vi "OceanOptics_30sec_img_while_scan_bare_Minimum.vi"() -> ()   [LabVIEW 2016]
uses:
  Maya2000 Typedefs/Maya2000 basic info.ctl
  C:/Program Files/Ocean Optics/OmniDriver/OOI_HOME/NETOmniDriver-NET40.dll
  Program Files/Ocean Optics/OmniDriver/OOI_HOME/NETOmniDriver-NET40.dll
  <vilib>/DAQmx/write.llb/DAQmx Write (Digital Bool 1Line 1Point).vi
  <vilib>/DAQmx/create/channels.llb/DAQmx Create Channel (DO-Digital Output).vi
  <vilib>/DAQmx/miscellaneous.llb/DAQmx Fill In Error Info.vi
panel:
  out "getExternalTriggerMode 2":i32
  in  "Trigger mode 2":i32
  in  "error in":errorcluster
  out "error out 2":errorcluster
  in  "Trigger":bool
  in  "Action B":bool
  out "getBufferCapacity":i32
  in  "read":bool
  in  "start":bool
  in  "abort":bool
  in  "stop":bool
  out "spectrum":cluster{"Y":dbl[], "Y":dbl[]}[](graph)
  out "getExternalTriggerMode":i32
  in  "Trigger mode":i32
  out "isFeatureSupportedDataBuffer":i16
  in  "clear":bool
  out "getNumberOfElements before readout":i32
  out "status":bool
  out "error out":errorcluster
  out "this maya":T1={"This instruments index"=0, "Name+SerialNumber"="MayaPro2000:MAYP111403", "Number Dark pixels"=8, "NumberOfPixels\nper spectrum"=2068, "NumberOf Maya2000 instrm."=2, "MaximumIntegrationTime\n[us]"=1600000000, "MinimumIntegrationTime\n[us]"=7200}
  in  "integration time [us]":i32=100000
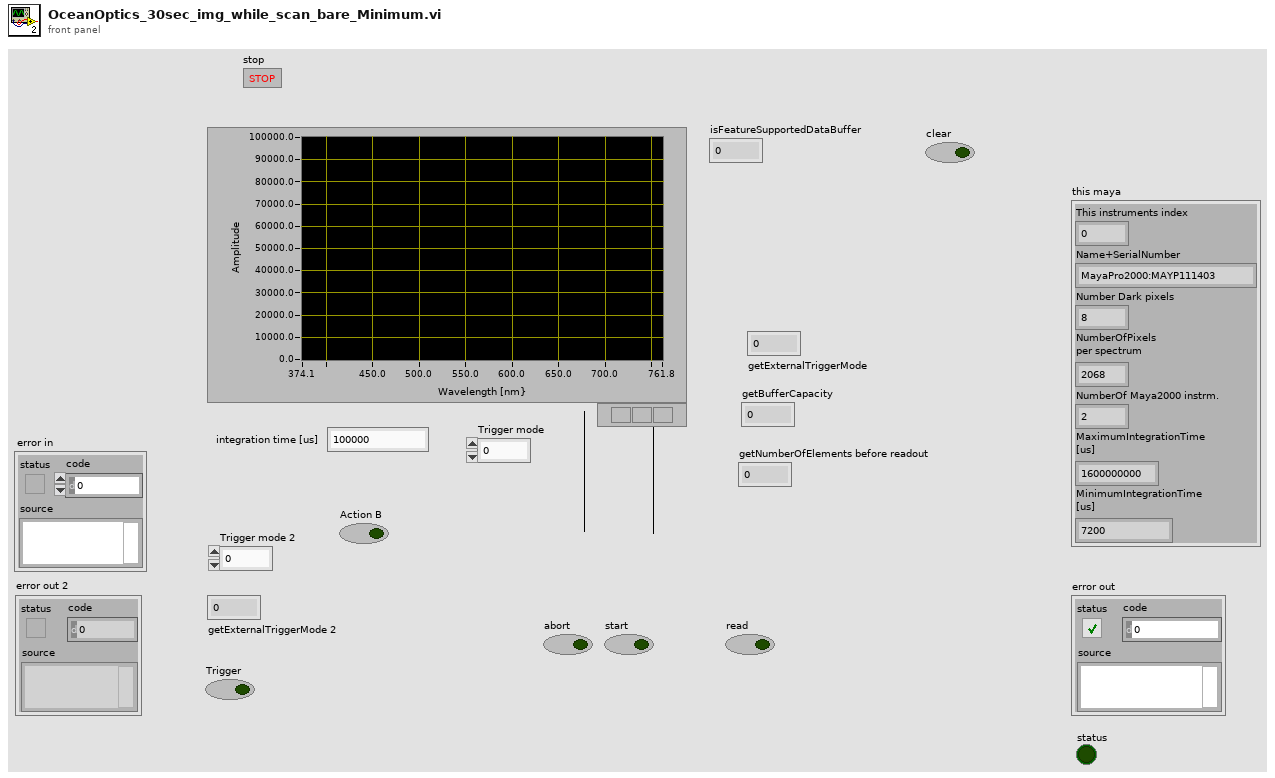
[diagram p1: front panel]
types:
  T1 = typedef "Maya2000 basic info.ctl" = cluster{"This instruments index":i32, "Name+SerialNumber":string, "Number Dark pixels":i32, "NumberOfPixels\nper spectrum":i32, "NumberOf Maya2000 instrm.":i32, "MaximumIntegrationTime\n[us]":i32, "MinimumIntegrationTime\n[us]":i32}
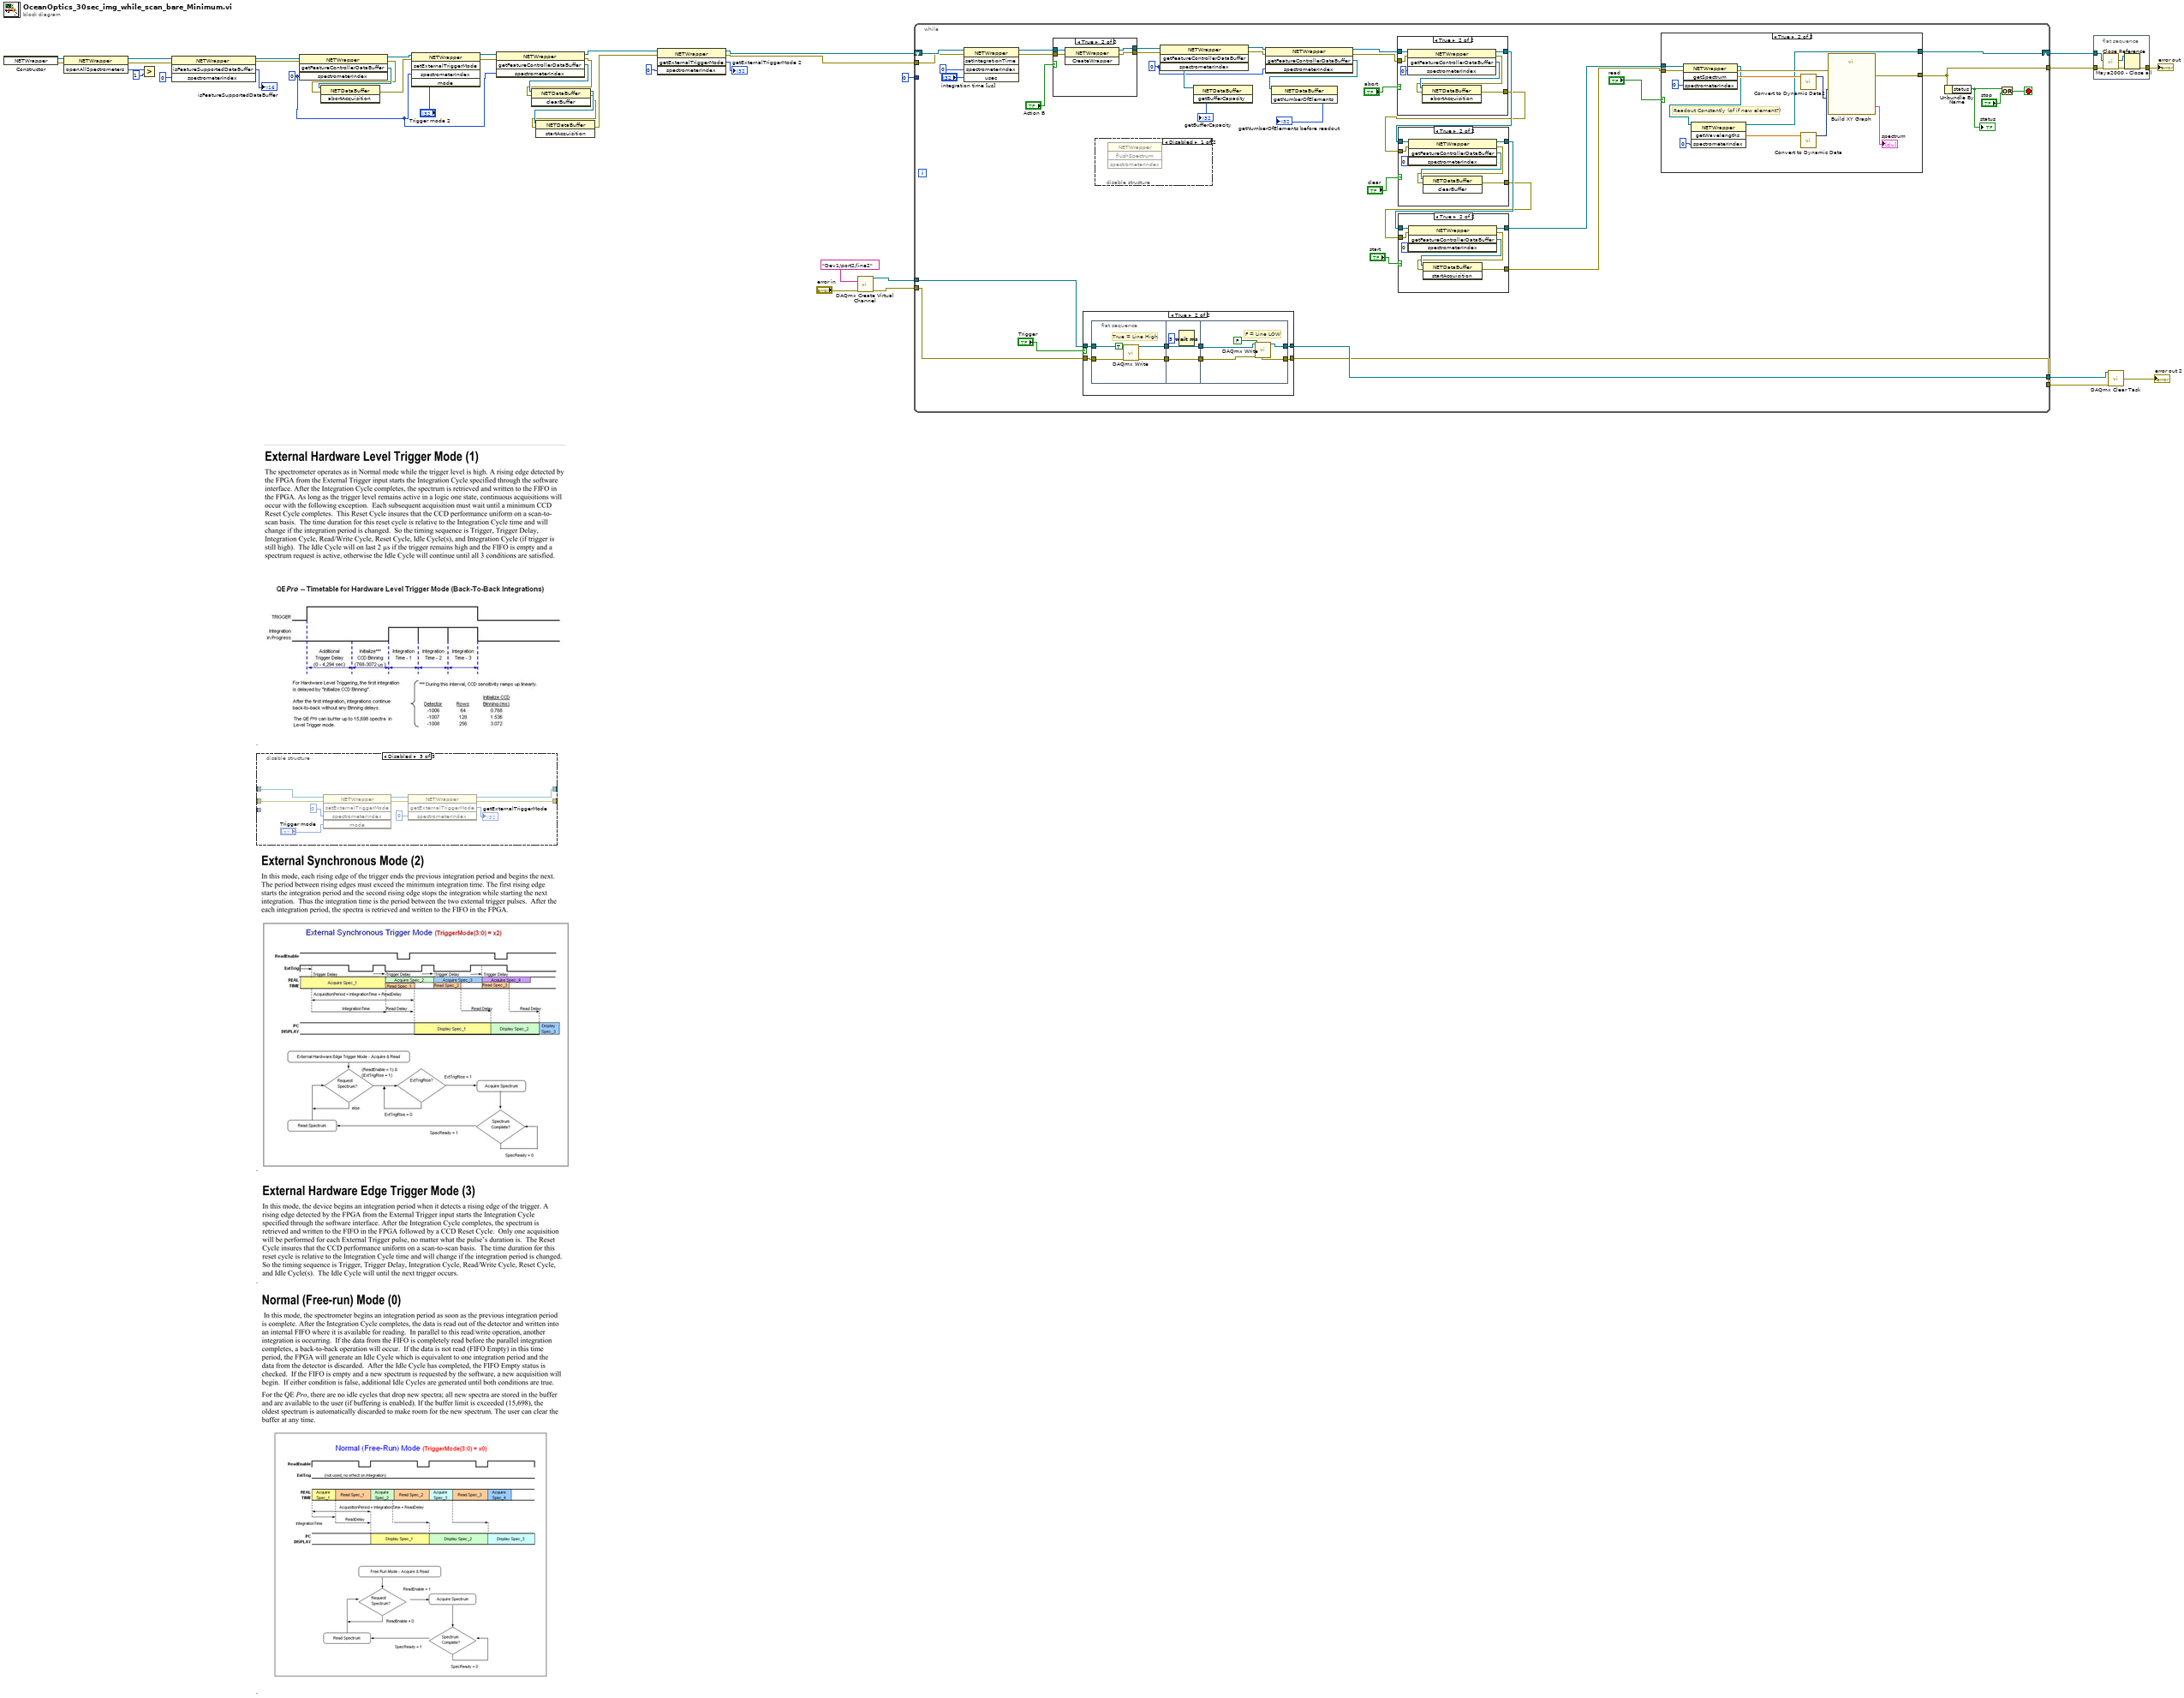
[diagram p0: block diagram]
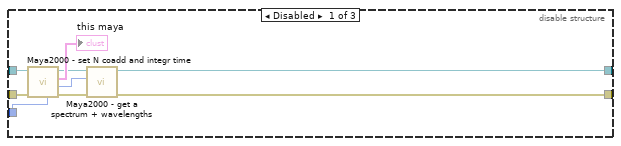
[diagram p9: hidden frame]
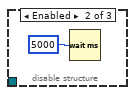
[diagram p10: hidden frame]
diagram:
  w7 = 0 ("spectrometerIndex")
  n1 = constructor class="NETWrapper"() -> (reference out=w34:refnum<k24>, error out=w33:errorcluster)  [unwired: 3 in, 1 out]
  n2 = invoke class="NETWrapper" method="openAllSpectrometers"(reference=w34, error in=w33) -> (reference out=w32:refnum<k24>, error out=w31:errorcluster, "openAllSpectrometers"=w30:i32)  [unwired: 1 in]
  n3 = Greater?(x=w30, y=1) -> ()  [unwired: 1 out]
  n4 = invoke class="NETWrapper" method="isFeatureSupportedDataBuffer"(reference=w32, error in=w31, "spectrometerIndex"=0) -> (reference out=w20:refnum<k24>, error out=w17:errorcluster, "isFeatureSupportedDataBuffer"=→"isFeatureSupportedDataBuffer":i16)  [unwired: 1 in, 1 out]
  n5 = disable-structure shown="Disabled" {
    disable-tunnel: _ -> [w50 _ w60]
    disable-tunnel: _ -> [w48 _ w53]
    disable-tunnel: [w43 _ w58] -> _
    disable-tunnel: [w41 _ w56] -> _
    disable-tunnel: _ -> [w40 _ _]
    frame Disabled {
      n6 = call "Maya2000 - set N coadd and integr time.vi"("Intgration time\n[us]"=w40, "error in (no error)"=w48, ".NET Refnum in"=w50) -> ("error out"=w45:errorcluster, "This instruments index"=w42:i32, "This Maya´\nbasic info"=→"this maya":T1, ".NET Refnum out"=w46:refnum<k24>, "numberOfScans\nToAverage"=w47:u32, "Maya2000 basic values"=w49:T1[])  [unwired: 3 in]
      n7 = call "Maya2000 - get a spectrum + wavelengths.vi"("error in (no error)"=w45, "This instrments index"=w42, ".NET Refnum in"=w46) -> ("error out"=w41:errorcluster, "Wavelengths"=w44:dbl[], ".NET Refnum out"=w43:refnum<k24>)  [unwired: 3 in, 3 out]
    }
    frame Enabled {
      n8 = Wait (ms)(milliseconds to wait=u32 5000) -> ()  [unwired: 1 out]
    }
    frame Disabled {
      n9 = invoke class="NETWrapper" method="setExternalTriggerMode"(reference=w60, error in=w53, "spectrometerIndex"=0, "mode"="Trigger mode") -> (reference out=w59:refnum<k24>, error out=w57:errorcluster)  [unwired: 1 in, 3 out]
      n10 = invoke class="NETWrapper" method="getExternalTriggerMode"(reference=w59, error in=w57, "spectrometerIndex"=0) -> (reference out=w58:refnum<k24>, error out=w56:errorcluster, "getExternalTriggerMode"=→"getExternalTriggerMode":i32)  [unwired: 1 in, 1 out]
    }
  }
  n11 = invoke class="NETWrapper" method="getFeatureControllerDataBuffer"(reference=w20, error in=w17, "spectrometerIndex"=w7) -> (reference out=w18:refnum<k24>, error out=w9:errorcluster, "getFeatureControllerDataBuffer"=w10:refnum<k24>)  [unwired: 1 in, 1 out]
  n12 = invoke class="NETDataBuffer" method="abortAcquisition"(reference=w10, error in=w9) -> (error out=w8:errorcluster)  [unwired: 1 in, 2 out]
  n13 = invoke class="NETWrapper" method="setExternalTriggerMode"(reference=w18, error in=w8, "spectrometerIndex"=w7, "mode"="Trigger mode 2") -> (reference out=w12:refnum<k24>, error out=w11:errorcluster)  [unwired: 1 in, 3 out]
  n14 = invoke class="NETWrapper" method="getFeatureControllerDataBuffer"(reference=w12, error in=w11, "spectrometerIndex"=w7) -> (reference out=w4:refnum<k24>, error out=w13:errorcluster, "getFeatureControllerDataBuffer"=w15:refnum<k24>)  [unwired: 1 in, 1 out]
  n15 = invoke class="NETDataBuffer" method="clearBuffer"(reference=w15, error in=w13) -> (reference out=w16:refnum<k24>, error out=w14:errorcluster)  [unwired: 1 in, 1 out]
  n16 = invoke class="NETDataBuffer" method="startAcquisition"(reference=w16, error in=w14) -> (error out=w3:errorcluster)  [unwired: 1 in, 2 out]
  n17 = invoke class="NETWrapper" method="getExternalTriggerMode"(reference=w4, error in=w3, "spectrometerIndex"=0) -> (reference out=w2:refnum<k24>, error out=w1:errorcluster, "getExternalTriggerMode"=→"getExternalTriggerMode 2":i32)  [unwired: 1 in, 1 out]
  n18 = call-poly <vilib>:"DAQmx Create Virtual Channel.vi"("lines"=tag "Dev1/port2/line2", "error in"="error in") -> ("task out"=w26:refnum<k21>, "error out"=w25:errorcluster)  [unwired: 12 in]
  n19 = while {
    tunnel: [w97] -> w38
    tunnel: 0 ("spectrometerIndex") -> [_]
    tunnel: w1 -> [w93]
    shift-right: [w100] -> w39
    shift-left: w2 -> [w94]
    tunnel: w26 -> [w82]
    tunnel: w25 -> [w81]
    tunnel: [w80] -> w23
    tunnel: [w79] -> w22
    stop <- w96 stop-if-true
    w74 = 0 ("spectrometerIndex")
    n20 = invoke class="NETWrapper" method="setIntegrationTime"(reference=w94, error in=w93, "spectrometerIndex"=0 ("mode"), "usec"="integration time [us]") -> (reference out=w84:refnum<k24>, error out=w83:errorcluster)  [unwired: 1 in, 3 out]
    n21 = case shown="True" "Action B" {
      tunnel: w84 -> [w143 w147]
      tunnel: [w143 w146] -> w87
      tunnel: w83 -> [w142 w145]
      tunnel: [w142 w144] -> w86
      frame False {
      }
      frame True {
        n22 = invoke class="NETWrapper" method="CreateWrapper"(reference=w147, error in=w145) -> (reference out=w146:refnum<k24>, error out=w144:errorcluster)  [unwired: 1 in, 1 out]
      }
    }
    n23 = case shown="True" "Trigger" {
      tunnel: w82 -> [w120 w124]
      tunnel: w81 -> [w119 w123]
      tunnel: [w120 w122] -> w80
      tunnel: [w119 w121] -> w79
      frame False {
      }
      frame True {
        n24 = flat-sequence {
          tunnel: w124 -> [w133]
          tunnel: w123 -> [w132]
          tunnel: [w131] -> w128
          tunnel: [w130] -> w127
          tunnel: w128 -> [w136]
          tunnel: w127 -> [w135]
          tunnel: [w136] -> w126
          tunnel: [w135] -> w125
          tunnel: [w139] -> w121
          tunnel: [w140] -> w122
          tunnel: w126 -> [w138]
          tunnel: w125 -> [w137]
          frame #0 {
            # "True = Line High"
            n25 = call-poly <vilib>:"DAQmx Write.vi"("task/channels in"=w133, "data"=TRUE, "error in"=w132) -> ("task out"=w131:refnum<k21>, "error out"=w130:errorcluster)  [unwired: 10 in, 1 out]
          }
          frame #1 {
            n26 = Wait (ms)(milliseconds to wait=u32 5) -> ()  [unwired: 1 out]
          }
          frame #2 {
            # "F = Line LOW"
            n27 = call-poly <vilib>:"DAQmx Write.vi"("task/channels in"=w138, "data"=FALSE, "error in"=w137) -> ("task out"=w140:refnum<k21>, "error out"=w139:errorcluster)  [unwired: 10 in, 1 out]
          }
        }
      }
    }
    n28 = disable-structure shown="Disabled" {
      frame Disabled {
        n29 = invoke class="NETWrapper" method="flushSpectrum"() -> ()  [unwired: 4 in, 4 out]
      }
      frame Enabled {
      }
    }
    n30 = invoke class="NETWrapper" method="getFeatureControllerDataBuffer"(reference=w87, error in=w86, "spectrometerIndex"=w74) -> (reference out=w76:refnum<k24>, error out=w75:errorcluster, "getFeatureControllerDataBuffer"=w92:refnum<k24>)  [unwired: 1 in, 1 out]
    n31 = invoke class="NETDataBuffer" method="getBufferCapacity"(reference=w92) -> ("getBufferCapacity"=→"getBufferCapacity":i32)  [unwired: 2 in, 2 out]
    n32 = invoke class="NETWrapper" method="getFeatureControllerDataBuffer"(reference=w76, error in=w75, "spectrometerIndex"=w74) -> (reference out=w73:refnum<k24>, error out=w72:errorcluster, "getFeatureControllerDataBuffer"=w77:refnum<k24>)  [unwired: 1 in, 1 out]
    n33 = invoke class="NETDataBuffer" method="getNumberOfElements"(reference=w77) -> ("getNumberOfElements"=→"getNumberOfElements before readout":i32)  [unwired: 2 in, 2 out]
    n34 = case shown="True" "abort" {
      tunnel: w73 -> [w163 w171]
      tunnel: [w163 w166] -> w67
      tunnel: [w164 w168] -> w64
      tunnel: w72 -> [w164 w167]
      frame False {
      }
      frame True {
        n35 = invoke class="NETWrapper" method="getFeatureControllerDataBuffer"(reference=w171, error in=w167, "spectrometerIndex"=0) -> (reference out=w166:refnum<k24>, error out=w169:errorcluster, "getFeatureControllerDataBuffer"=w170:refnum<k24>)  [unwired: 1 in, 1 out]
        n36 = invoke class="NETDataBuffer" method="abortAcquisition"(reference=w170, error in=w169) -> (error out=w168:errorcluster)  [unwired: 1 in, 2 out]
      }
    }
    n37 = case shown="True" "clear" {
      tunnel: w67 -> [w110 w118]
      tunnel: [w110 w113] -> w66
      tunnel: [w111 w115] -> w65
      tunnel: w64 -> [w111 w114]
      frame False {
      }
      frame True {
        n38 = invoke class="NETWrapper" method="getFeatureControllerDataBuffer"(reference=w118, error in=w114, "spectrometerIndex"=0) -> (reference out=w113:refnum<k24>, error out=w116:errorcluster, "getFeatureControllerDataBuffer"=w117:refnum<k24>)  [unwired: 1 in, 1 out]
        n39 = invoke class="NETDataBuffer" method="clearBuffer"(reference=w117, error in=w116) -> (error out=w115:errorcluster)  [unwired: 1 in, 2 out]
      }
    }
    n40 = case shown="True" "start" {
      tunnel: w66 -> [w101 w109]
      tunnel: [w101 w108] -> w68
      tunnel: [w102 w105] -> w63
      tunnel: w65 -> [w102 w104]
      frame False {
      }
      frame True {
        n41 = invoke class="NETWrapper" method="getFeatureControllerDataBuffer"(reference=w109, error in=w104, "spectrometerIndex"=0) -> (reference out=w108:refnum<k24>, error out=w106:errorcluster, "getFeatureControllerDataBuffer"=w107:refnum<k24>)  [unwired: 1 in, 1 out]
        n42 = invoke class="NETDataBuffer" method="startAcquisition"(reference=w107, error in=w106) -> (error out=w105:errorcluster)  [unwired: 1 in, 2 out]
      }
    }
    n43 = case shown="True" "read" {
      tunnel: [w148 w150] -> w100
      tunnel: [w149 w162] -> w97
      tunnel: w68 -> [w148 w154]
      tunnel: w63 -> [w149 w153]
      frame False {
      }
      frame True {
        # "Readout Constantly (of if new element?)"
        n44 = invoke class="NETWrapper" method="getSpectrum"(reference=w154, error in=w153, "spectrometerIndex"=0) -> (reference out=w151:refnum<k24>, error out=w152:errorcluster, "getSpectrum"=w156:dbl[])  [unwired: 1 in, 1 out]
        n45 = invoke class="NETWrapper" method="getWavelengths"(reference=w151, "spectrometerIndex"=0) -> (reference out=w150:refnum<k24>, "getWavelengths"=w160:dbl[])  [unwired: 2 in, 2 out]
        n46 = call "Convert to Dynamic Data2"("Array"=w156) -> ("Dynamic Data Type"=w157:dynamicdata)  [unwired: 3 in]
        n47 = call "Convert to Dynamic Data"("Array"=w160) -> ("Dynamic Data Type"=w158:dynamicdata)  [unwired: 3 in]
        n48 = call "Build XY Graph"("error in (no error)"=w152, "Y Input"=w157, "X Input"=w158) -> ("error out"=w162:errorcluster, "XY Graph"=→"spectrum":cluster{"X":dbl[], "Y":dbl[]}[])  [unwired: 7 in]
      }
    }
    n49 = Unbundle By Name(w97) -> ("status"=w89:bool)
    "status" <- w89
    n50 = Or(x=w89, y="stop") -> (x .or. y?=w96:bool)
  }
  n51 = flat-sequence {
    tunnel: w39 -> [w176]
    tunnel: w38 -> [w175]
    tunnel: [w174] -> w37
    frame #0 {
      n52 = call "Maya2000 - Close all.vi"("error in (no error)"=w175, "Maya reference in"=w176) -> ("error out"=w173:errorcluster, ".NET Refnum out"=w172:refnum<k24>)  [unwired: 8 in]
      n53 = Close Reference(reference=w172, error in (no error)=w173) -> (error out=w174:errorcluster)
    }
  }
  n54 = call <vilib>:"DAQmx Clear Task.vi"("task in"=w23, "error in"=w22) -> ("error out"=→"error out 2":errorcluster)  [unwired: 13 in]
  "error out" <- w37
